vi "Example Three Stage.vi"() -> ()   [LabVIEW 2019]
uses:
  Class/Controller/Controller.lvclass
  <vilib>/Platform/TimedLoop/XDataNode/timing_clust.ctl
  <vilib>/Platform/TimedLoop/XDataNode/nitl_modes.ctl
  <vilib>/Platform/TimedLoop/XDataNode/wakeup.ctl
  <vilib>/platform/TimedLoop/XDataNode/XDataNode.xnode
  <vilib>/Platform/TimedLoop/XDataNode/XDNodeRunTimeDep.lvlib
panel:
  in  "Tab Control 3":enum32{"Motion", "Settings"}(tab)
  in  "Zero Output 3":bool
  in  "Go to Home 3":bool
  in  "Scan Right 3":bool
  in  "Scan Left 3":bool
  in  "Continue 3":bool
  in  "Stop 3":bool
  in  "Make Step Right 3":bool
  in  "Step Size \n[selected units] 3":dbl=1.0 format="%#.2f"
  in  "Make Step Left 3":bool
  in  "Desired Speed \n[1µm/s or 0,01deg /s] 3":dbl=10000.0 format="%#.2f"
  in  "Desired Position \n[selected units] 3":dbl format="%#.2f"
  in  "Find Index 3":bool
  in  "Reset 3":bool
  out "Desired Position\n[selected units] 3":dbl
  out "Encoder position \n[selected units] 3":dbl
  out "Waveform Chart 3":dbl(graph)=-0.078
  out "Status Info 3":T1
  out "StatusBits 3":T2
  in  "Working Units 3":string(combo)="1000000"
  in  "Axis Resolution 3":string(combo)="312,5"
  in  "Axis Letter 3":string="Z"
  in  "Tab Control 2":enum32{"Motion", "Settings"}(tab)
  in  "Zero Output 2":bool
  in  "Go to Home 2":bool
  in  "Scan Right 2":bool
  in  "Scan Left 2":bool
  in  "Continue 2":bool
  in  "Stop 2":bool
  in  "Make Step Right 2":bool
  in  "Step Size \n[selected units] 2":dbl=1.0 format="%#.2f"
  in  "Make Step Left 2":bool
  in  "Desired Speed \n[1µm/s or 0,01deg /s] 2":dbl=10000.0 format="%#.2f"
  in  "Desired Position \n[selected units] 2":dbl format="%#.2f"
  in  "Find Index 2":bool
  in  "Reset 2":bool
  out "Desired Position\n[selected units] 2":dbl
  out "Encoder position \n[selected units] 2":dbl
  out "Waveform Chart 2":dbl(graph)=-0.078
  out "Status Info 2":T1
  out "StatusBits 2":T2
  out "Desired Position\n[selected units]":dbl
  out "Encoder position \n[selected units]":dbl
  in  "Tab Control":enum32{"Motion", "Settings"}(tab)
  in  "Zero Output":bool
  in  "Go to Home":bool
  in  "Scan Right":bool
  in  "Scan Left":bool
  in  "Continue":bool
  in  "Stop":bool
  in  "Make Step Right":bool
  in  "Step Size \n[selected units]":dbl=1.0 format="%#.2f"
  in  "Make Step Left":bool
  in  "Desired Speed \n[1µm/s or 0,01deg /s]":dbl=10000.0 format="%#.2f"
  in  "Desired Position \n[selected units]":dbl format="%#.2f"
  in  "Find Index":bool
  in  "Reset":bool
  out "error out":errorcluster
  in  "Working Units 2":string(combo)="1000000"
  in  "Working Units":string(combo)="1000000"
  out "StatusBits":T2
  out "Status Info":T1
  in  "Axis Resolution 2":string(combo)="312,5"
  in  "Axis Letter 2":string="Y"
  in  "Axis Resolution":string(combo)="312,5"
  in  "Axis Letter":string="X"
  in  "Baudrate":u32=9600
  in  "COM Port":refnum<visa-resource-name>
  in  "Controller.lvclass":refnum<class "Controller.lvclass">
  out "Waveform Chart":dbl(graph)=-0.078
  in  "STOP PROGRAM":bool
  # "Visualization"
  # "Extra information"
  # "READ ME FIRST"
  # "Configuration"
  # "Stage 1"
  # "Driver 1"
  # "Stage 1"
  # "How to run:"
  # "BEFORE RUNNING:"
  # "1, Select COM Port"
  # "2. Select baudrate"
  # "3. For each axis:"
  # "3.1 Specify correct axis name (1 letter)"
  # "3.2 Specify correct resolution"
  # "4. Run VI"
  # "WHEN RUNNING, YOU HAVE TO FIRST PUSH \"FIND INDEX\" FOR EACH STAGE.\nThe stages will start moving and find its position. After that you can control the stages"
  # "Stage 2"
  # "NOTES: Do this only the first time"
  # "1. Replace the settings_default.txt file with\nthe file we provided on a USB stick."
  # "2.    Make sure there are no comments in the\nsettings_default.txt file. ONLY lines like: \"X:DPOS=100\" so NO \"%\" in front or at the end of the line."
  # "Position Information"
  # "Stage 3"
  # "3.  In your settings_default.txt file:\nEvery line that contains SSPD or MSPD: multiply that value with:\n - 1000 for a lineair stage \n - 100 for a rotating stage"
  # "STOP BUTTON"
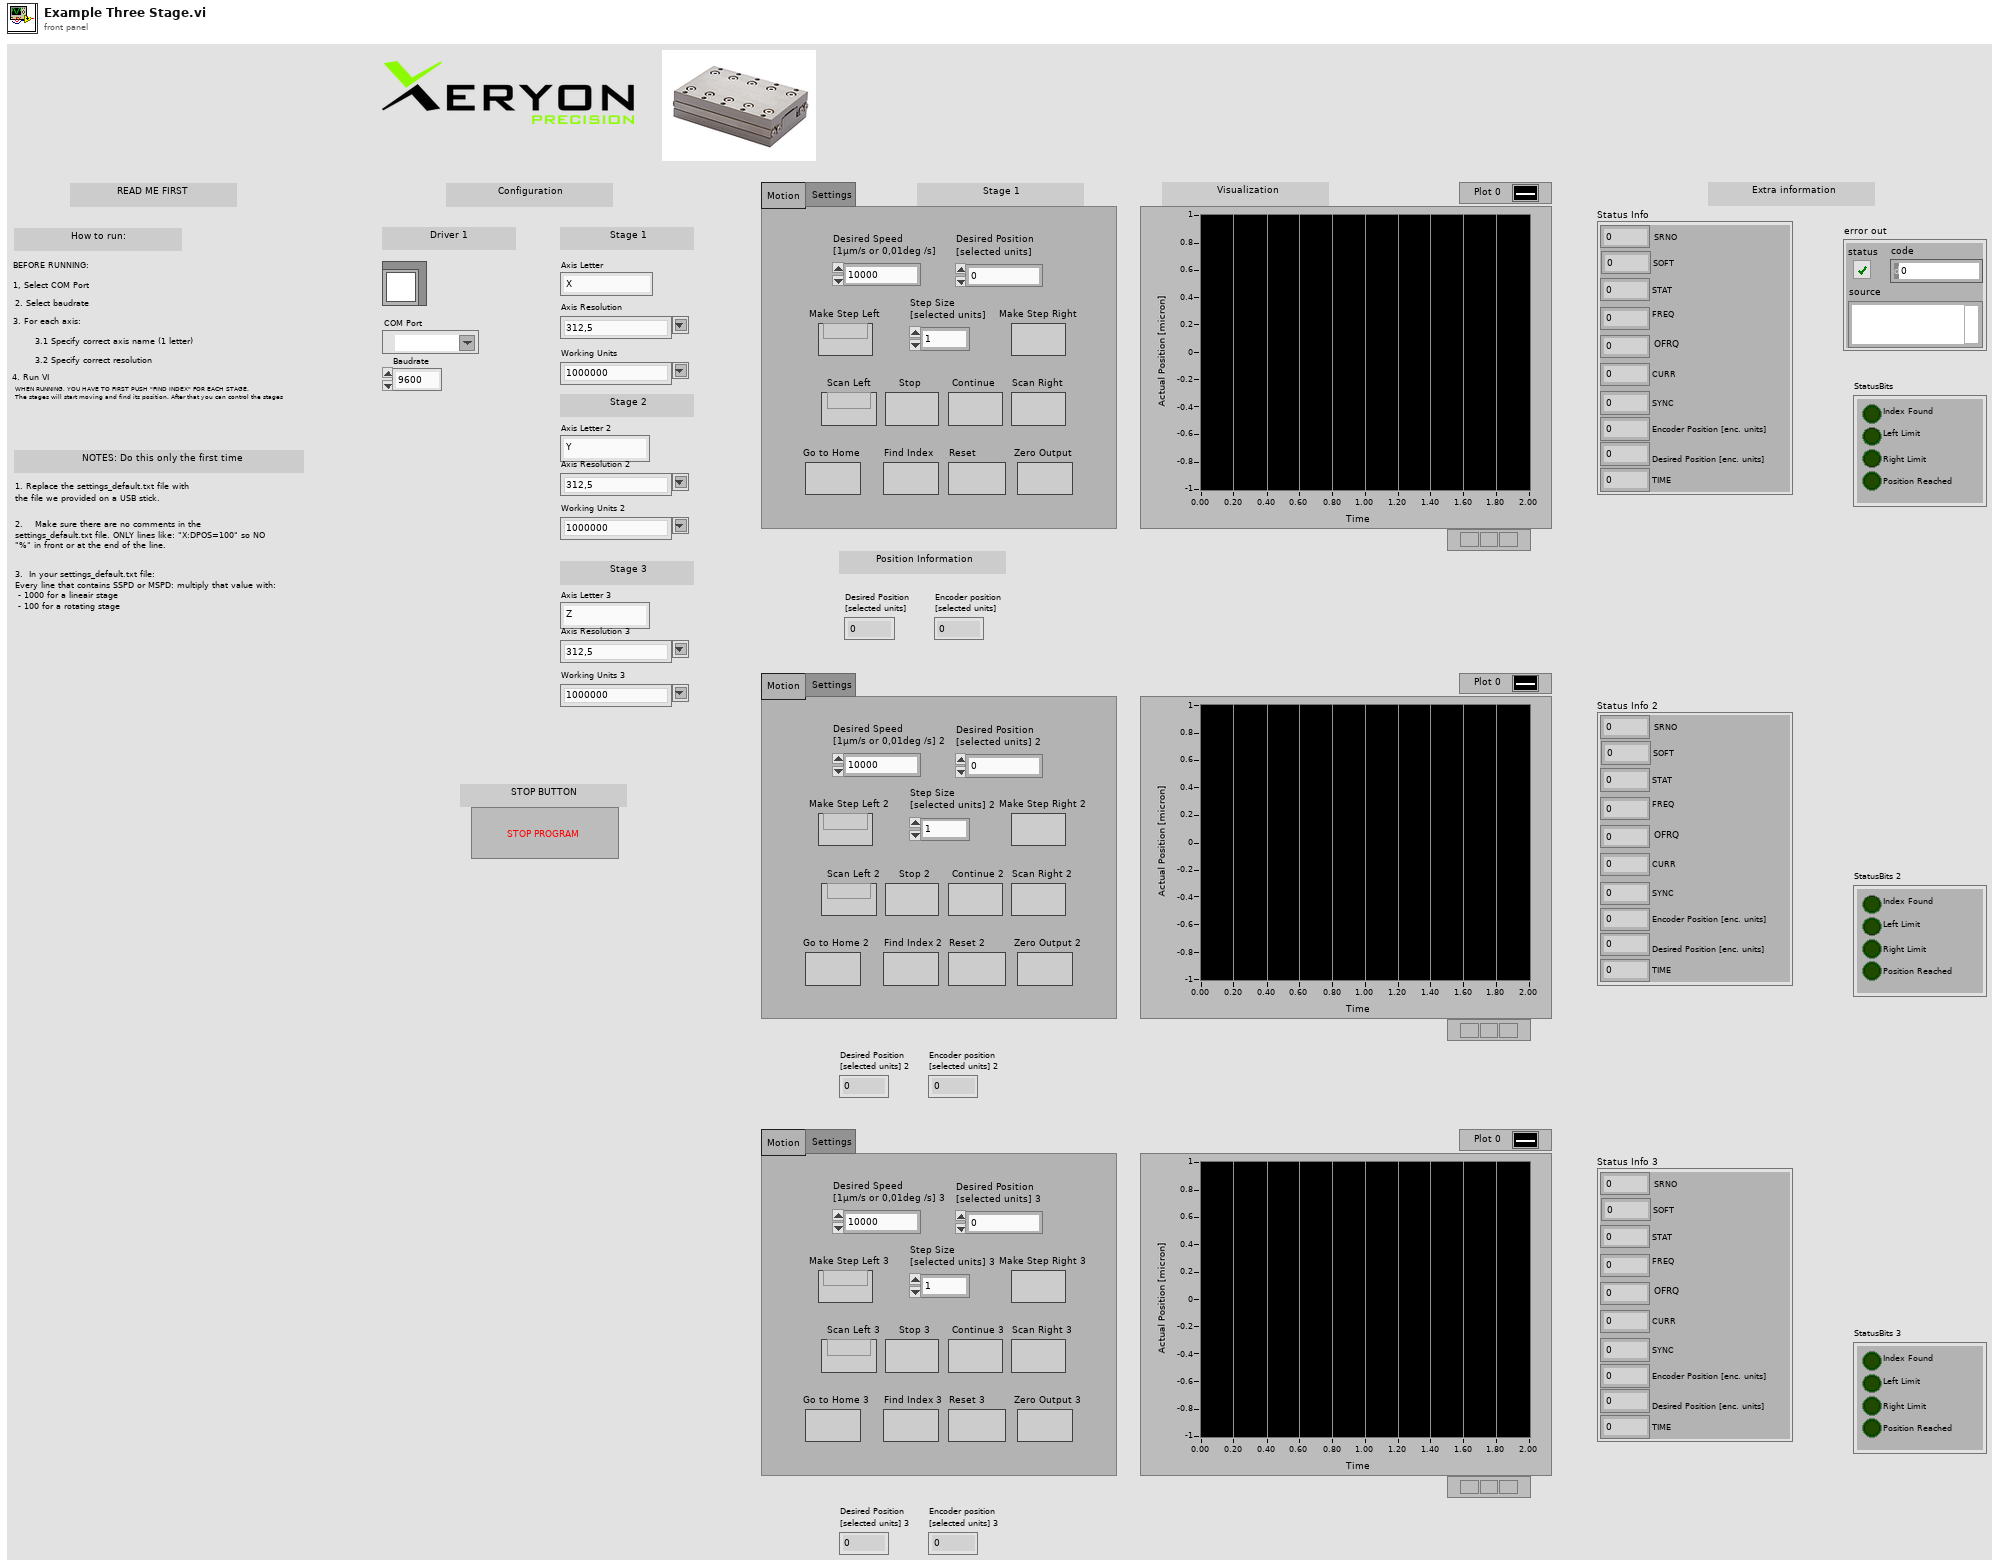
[diagram p1: front panel]
types:
  T1 = cluster{"SRNO":dbl, "SOFT":dbl, "STAT":dbl, "FREQ":dbl, "OFRQ":dbl, "CURR":dbl, "SYNC":dbl, "Encoder Position [enc. units]":dbl, "Desired Position [enc. units]":dbl, "TIME":dbl}
  T2 = cluster{"Index Found":bool, "Left Limit":bool, "Right Limit":bool, "Position Reached":bool}
  T3 = typedef "XDNodeRunTimeDep.lvlib/timing_clust.ctl" = cluster{"Expected End [f-1]":u64, "Actual End [f-1]":u64, "Finished Late? [f-1]":bool, "Expected End [i-1]":u64, "Actual End [i-1]":u64, "Finished Late? [i-1]":bool, "Expected Start [i]":u64, "Actual Start [i]":u64, "Expected Start [f]":u64, "Actual Start [f]":u64, "Source Name":string, "Structure Name":string, "Period":i64, "Deadline":i64, "Offset":i64, "Start":i64, "Priority":i32, "Timeout":i32, "Mode":T4, "Wakeup Reason":T5, "Error":errorcluster, "Source Type":string, "Secondary Source Type":string, "Global End Time":u64, "Global Start Time":u64, "Frame Duration":u64, "Iteration Duration":u64, "Assigned CPU":i32, "I/O Scan Engine Mode":u32}
  T4 = typedef "XDNodeRunTimeDep.lvlib/nitl_modes.ctl" = enum32{"No Change", "Process missed periods, maintain original phase", "Discard missed periods, maintain original phase", "Process missed periods, ignore original phase", "Discard missed periods, ignore original phase"}
  T5 = typedef "XDNodeRunTimeDep.lvlib/wakeup.ctl" = enum32{"Normal", "Aborted", "Asynchronous wakeup", "Timing source error", "Timed loop error", "Timeout"}
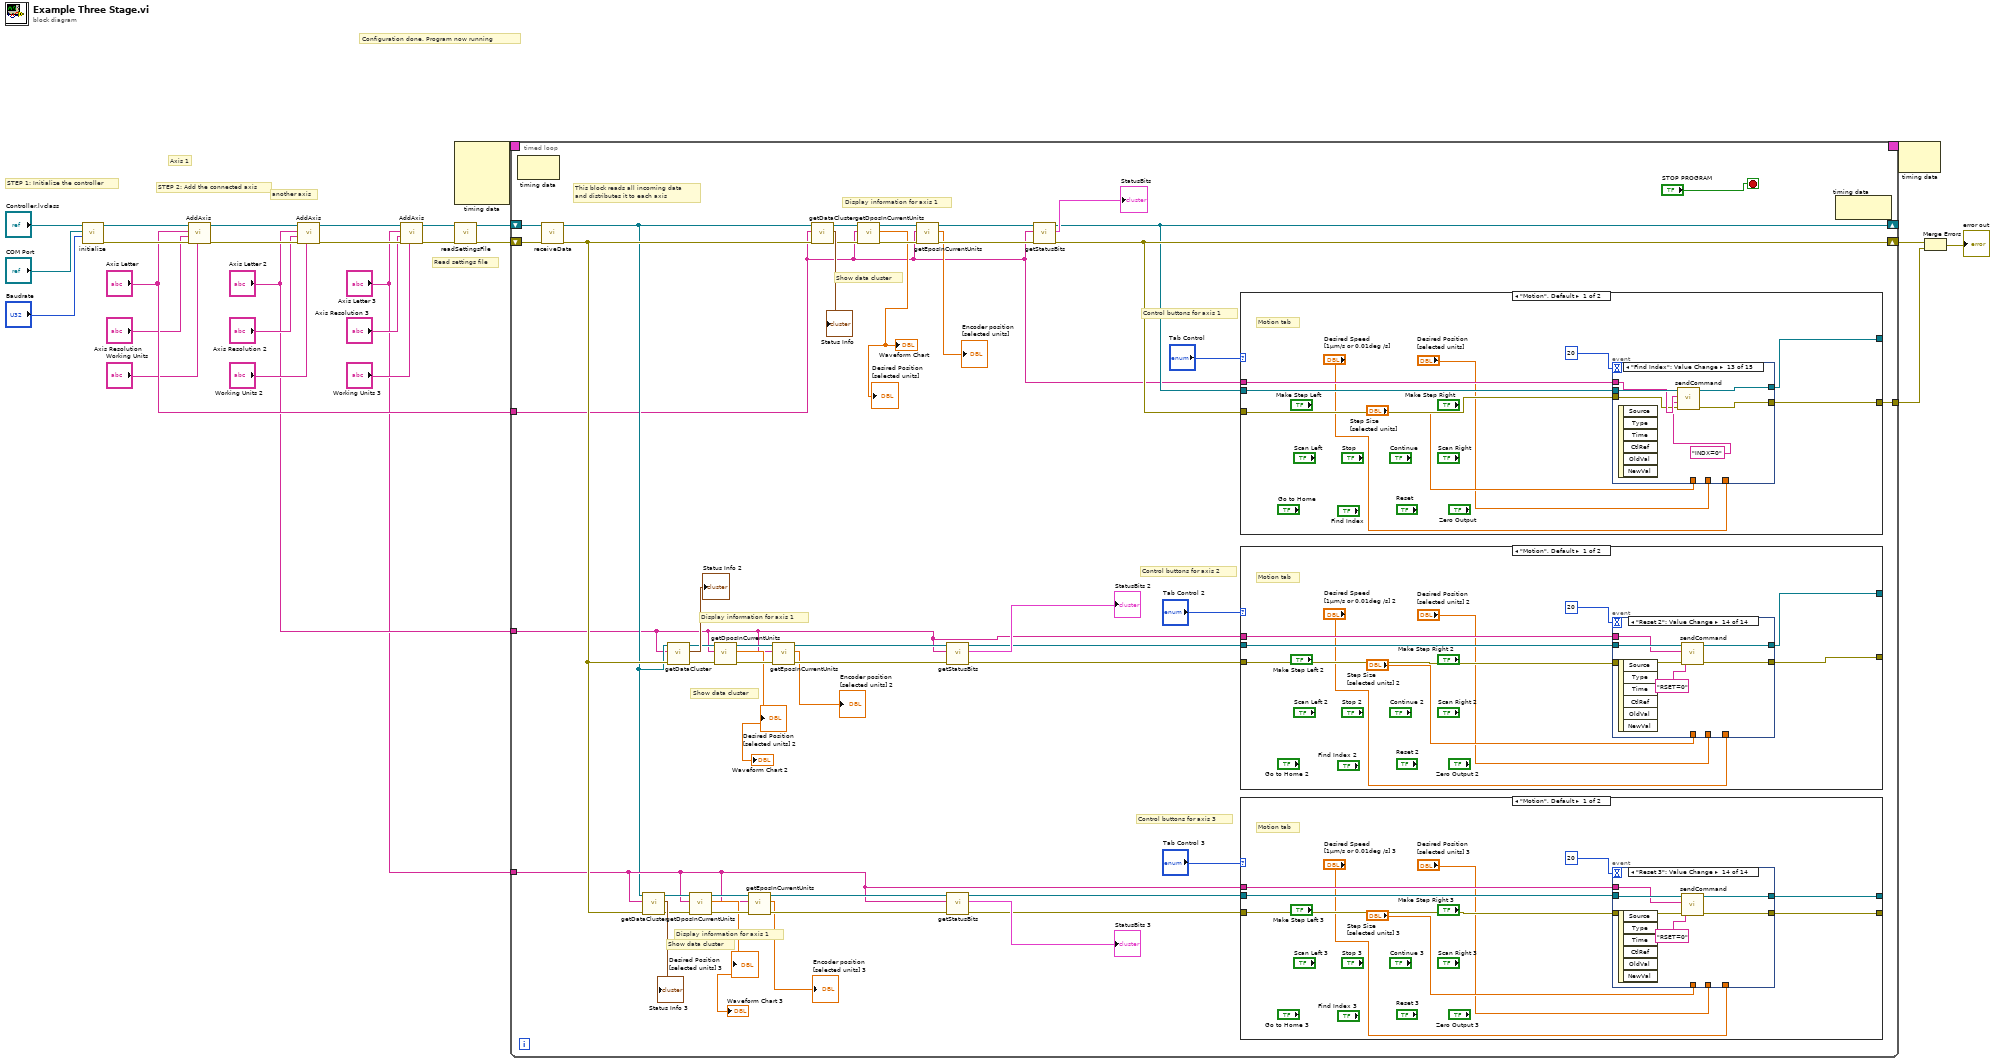
[diagram p0: block diagram]
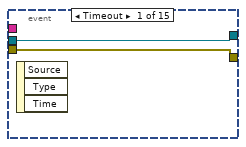
[diagram p2: hidden frame]
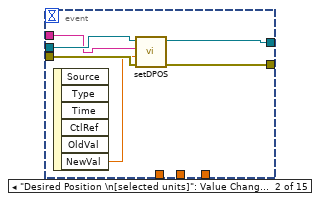
[diagram p3: hidden frame]
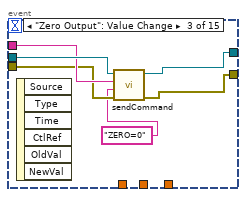
[diagram p4: hidden frame]
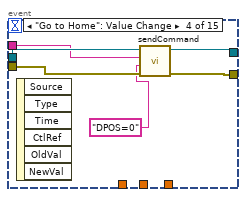
[diagram p5: hidden frame]
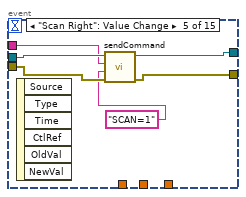
[diagram p6: hidden frame]
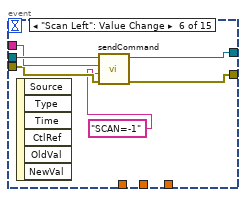
[diagram p7: hidden frame]
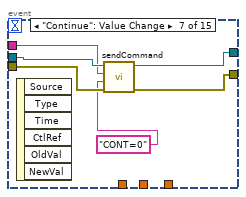
[diagram p8: hidden frame]
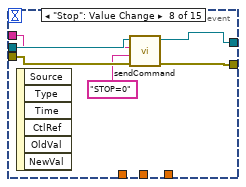
[diagram p9: hidden frame]
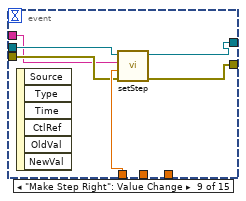
[diagram p10: hidden frame]
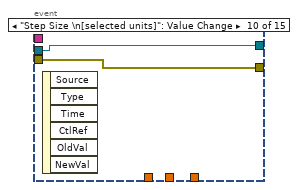
[diagram p11: hidden frame]
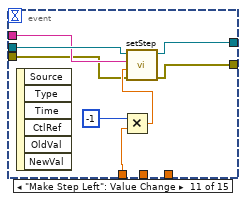
[diagram p12: hidden frame]
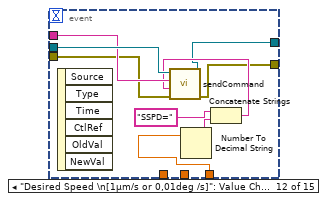
[diagram p13: hidden frame]
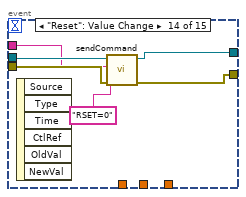
[diagram p14: hidden frame]
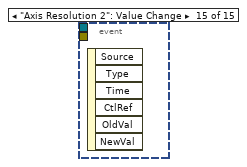
[diagram p15: hidden frame]
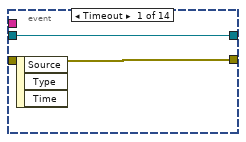
[diagram p17: hidden frame]
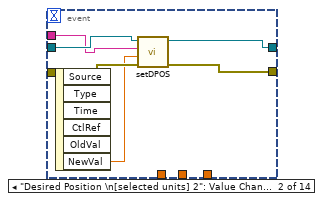
[diagram p18: hidden frame]
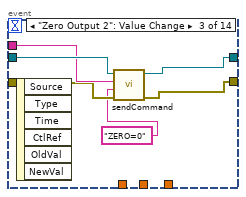
[diagram p19: hidden frame]
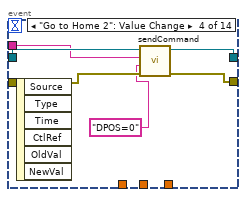
[diagram p20: hidden frame]
diagram:
  # "Axis 1"
  # "Configuration done. Program now running"
  # "Read settings file"
  # "another axis"
  # "STEP 2: Add the connected axis"
  # "STEP 1: Initialize the controller"
  n1 = call-dynamic "initialize.vi"("Baudrate"="Baudrate", "COM Port"="COM Port", "Controller in"="Controller.lvclass") -> ("error out"=w26:errorcluster, "Controller out"=w27:refnum<class "Controller.lvclass">)  [unwired: 7 in]
  n2 = call-dynamic "AddAxis.vi"("Units"="Working Units", "error in (no error)"=w26, "Encoder Resolution"="Axis Resolution", "Axis Letter"="Axis Letter", "Controller in"=w27) -> ("error out"=w24:errorcluster, "Controller out"=w25:refnum<class "Controller.lvclass">)  [unwired: 5 in]
  n3 = call-dynamic "AddAxis.vi"("Units"="Working Units 2", "error in (no error)"=w24, "Encoder Resolution"="Axis Resolution 2", "Axis Letter"="Axis Letter 2", "Controller in"=w25) -> ("error out"=w11:errorcluster, "Controller out"=w12:refnum<class "Controller.lvclass">)  [unwired: 5 in]
  n4 = call-dynamic "AddAxis.vi"("Units"="Working Units 3", "error in (no error)"=w11, "Encoder Resolution"="Axis Resolution 3", "Axis Letter"="Axis Letter 3", "Controller in"=w12) -> ("error out"=w19:errorcluster, "Controller out"=w21:refnum<class "Controller.lvclass">)  [unwired: 5 in]
  n5 = node-c288() -> (w9:T3)  [unwired: 4 in]
  n6 = call-dynamic "readSettingsFile.vi"("error in (no error)"=w19, "Controller in"=w21) -> ("error out"=w18:errorcluster, "Controller out"=w20:refnum<class "Controller.lvclass">)  [unwired: 8 in]
  n7 = timed-loop {
    shift-right: [w29] -> _
    shift-left: w20 -> [w75]
    tunnel: "Axis Letter" -> [w28]
    shift-right: [w61] -> w7
    shift-left: w18 -> [w64]
    timing: w9 -> [_]
    timing-out: [_] -> w8
    tunnel: [w60] -> w6
    tunnel: "Axis Letter 2" -> [w30]
    tunnel: "Axis Letter 3" -> [w32]
    stop <- "STOP PROGRAM" stop-if-true
    # "Control buttons for axis 3"
    # "Display information for axis 1"
    # "Show data cluster"
    # "Control buttons for axis 2"
    # "Display information for axis 1"
    # "Show data cluster"
    # "Control buttons for axis 1"
    # "Display information for axis 1"
    # "Show data cluster"
    # "This block reads all incoming data\nand distributes it to each axis"
    n8 = node-c288() -> ()  [unwired: 1 in, 1 out]
    n9 = call-dynamic "receiveData.vi"("error in (no error)"=w64, "Controller in"=w75) -> ("error out"=w33:errorcluster, "Controller out"=w31:refnum<class "Controller.lvclass">)  [unwired: 7 in, 1 out]
    n10 = call-dynamic "getDataCluster.vi"("error in (no error)"=w33, "Axis Letter"=w32, "Controller in"=w31) -> ("error out"=w41:errorcluster, "Information"=→"Status Info 3":T1, "Controller out"=w44:refnum<class "Controller.lvclass">)  [unwired: 6 in]
    n11 = call-dynamic "getDataCluster.vi"("error in (no error)"=w33, "Axis Letter"=w30, "Controller in"=w31) -> ("error out"=w54:errorcluster, "Information"=→"Status Info 2":T1, "Controller out"=w57:refnum<class "Controller.lvclass">)  [unwired: 6 in]
    n12 = call-dynamic "getDposInCurrentUnits.vi"("error in (no error)"=w41, "Axis Letter"=w32, "Controller in"=w44) -> ("error out"=w40:errorcluster, "DPOS In Current Units"=→"Waveform Chart 3" →"Desired Position\n[selected units] 3":dbl, "Controller out"=w43:refnum<class "Controller.lvclass">)  [unwired: 6 in]
    n13 = call-dynamic "getDposInCurrentUnits.vi"("error in (no error)"=w54, "Axis Letter"=w30, "Controller in"=w57) -> ("error out"=w53:errorcluster, "DPOS In Current Units"=→"Waveform Chart 2" →"Desired Position\n[selected units] 2":dbl, "Controller out"=w56:refnum<class "Controller.lvclass">)  [unwired: 6 in]
    n14 = call-dynamic "getEposInCurrentUnits.vi"("error in (no error)"=w40, "Axis Letter"=w32, "Controller in"=w43) -> ("error out"=w39:errorcluster, "EPOS In Current Units"=→"Encoder position \n[selected units] 3":dbl, "Controller out"=w42:refnum<class "Controller.lvclass">)  [unwired: 6 in]
    n15 = call-dynamic "getEposInCurrentUnits.vi"("error in (no error)"=w53, "Axis Letter"=w30, "Controller in"=w56) -> ("error out"=w52:errorcluster, "EPOS In Current Units"=→"Encoder position \n[selected units] 2":dbl, "Controller out"=w55:refnum<class "Controller.lvclass">)  [unwired: 6 in]
    n16 = call-dynamic "getDataCluster.vi"("error in (no error)"=w33, "Axis Letter"=w28, "Controller in"=w31) -> ("error out"=w69:errorcluster, "Information"=→"Status Info":T1, "Controller out"=w72:refnum<class "Controller.lvclass">)  [unwired: 6 in]
    n17 = call-dynamic "getDposInCurrentUnits.vi"("error in (no error)"=w69, "Axis Letter"=w28, "Controller in"=w72) -> ("error out"=w68:errorcluster, "DPOS In Current Units"=→"Waveform Chart" →"Desired Position\n[selected units]":dbl, "Controller out"=w71:refnum<class "Controller.lvclass">)  [unwired: 6 in]
    n18 = call-dynamic "getEposInCurrentUnits.vi"("error in (no error)"=w68, "Axis Letter"=w28, "Controller in"=w71) -> ("error out"=w67:errorcluster, "EPOS In Current Units"=→"Encoder position \n[selected units]":dbl, "Controller out"=w70:refnum<class "Controller.lvclass">)  [unwired: 6 in]
    n19 = call-dynamic "getStatusBits.vi"("error in (no error)"=w52, "Axis Letter"=w30, "Controller in"=w55) -> ("error out"=w47:errorcluster, "StatusBits"=→"StatusBits 2":T2, "Controller out"=w48:refnum<class "Controller.lvclass">)  [unwired: 6 in]
    n20 = call-dynamic "getStatusBits.vi"("error in (no error)"=w39, "Axis Letter"=w32, "Controller in"=w42) -> ("error out"=w34:errorcluster, "StatusBits"=→"StatusBits 3":T2, "Controller out"=w35:refnum<class "Controller.lvclass">)  [unwired: 6 in]
    n21 = call-dynamic "getStatusBits.vi"("error in (no error)"=w67, "Axis Letter"=w28, "Controller in"=w70) -> ("error out"=w61:errorcluster, "StatusBits"=→"StatusBits":T2, "Controller out"=w29:refnum<class "Controller.lvclass">)  [unwired: 6 in]
    n22 = case shown="\"Motion\", Default" "Tab Control" {
      tunnel: w29 -> [w86 w168]
      tunnel: w61 -> [w85 w169]
      tunnel: [w84 w168] -> _
      tunnel: [w83 w169] -> w60
      tunnel: w28 -> [w81 _]
      frame "Motion", Default {
        # "Motion tab"
        n23 = event shown="[12] \"Find Index\": Value Change" {
          selector: _ -> [_ _ _ _ _ _ _ _ _ _ _ _ _ _ _]
          dyn-events: _ -> [_ _ _ _ _ _ _ _ _ _ _ _ _ _ _]
          timeout: 20 -> [_ _ _ _ _ _ _ _ _ _ _ _ _ _ _]
          tunnel: w86 -> [w88 w94 w100 w106 w112 w118 w124 w130 w134 w138 w144 w155 w161 w167 _]
          tunnel: w85 -> [w87 w93 w98 w104 w110 w116 w122 w128 w135 w137 w141 w153 w159 w166 _]
          tunnel: [w88 w91 w96 w101 w108 w114 w120 w126 w132 w138 w139 w147 w157 w163 _] -> w84
          tunnel: [w87 w92 w97 w103 w109 w115 w121 w127 w131 w137 w140 w148 w158 w162 _] -> w83
          tunnel: w81 -> [_ w89 w99 w105 w111 w117 w123 w129 w133 _ w143 w154 w160 w165 _]
          tunnel: "Step Size \n[selected units]" -> [_ _ _ _ _ _ _ _ w136 _ w145 _ _ _ _]
          tunnel: "Desired Position \n[selected units]" -> [_ _ _ _ _ _ _ _ _ _ _ _ _ _ _]
          tunnel: "Desired Speed \n[1µm/s or 0,01deg /s]" -> [_ _ _ _ _ _ _ _ _ _ _ w152 _ _ _]
          event Timeout {
            n24 = event-data() -> ()  [unwired: 1 in, 3 out]
          }
          event "Desired Position \n[selected units]": Value Change {
            n25 = event-data() -> ("NewVal"=w90:dbl)  [unwired: 1 in, 5 out]
            n26 = call-dynamic "setDPOS.vi"("error in (no error)"=w93, "DPOS In Current Units"=w90, "Axis Letter"=w89, "Controller in"=w94) -> ("error out"=w92:errorcluster, "Controller out"=w91:refnum<class "Controller.lvclass">)  [unwired: 6 in]
          }
          event "Zero Output": Value Change {
            n27 = event-data() -> ()  [unwired: 1 in, 6 out]
            n28 = call-dynamic "sendCommand.vi"("error in (no error)"=w98, "Value"="ZERO=0", "Command"=w99, "Controller in"=w100) -> ("error out"=w97:errorcluster, "Controller out"=w96:refnum<class "Controller.lvclass">)  [unwired: 6 in]
          }
          event "Go to Home": Value Change {
            n29 = event-data() -> ()  [unwired: 1 in, 6 out]
            n30 = call-dynamic "sendCommand.vi"("error in (no error)"=w104, "Value"="DPOS=0", "Command"=w105, "Controller in"=w106) -> ("error out"=w103:errorcluster, "Controller out"=w101:refnum<class "Controller.lvclass">)  [unwired: 6 in]
          }
          event "Scan Right": Value Change {
            n31 = event-data() -> ()  [unwired: 1 in, 6 out]
            n32 = call-dynamic "sendCommand.vi"("error in (no error)"=w110, "Value"="SCAN=1", "Command"=w111, "Controller in"=w112) -> ("error out"=w109:errorcluster, "Controller out"=w108:refnum<class "Controller.lvclass">)  [unwired: 6 in]
          }
          event "Scan Left": Value Change {
            n33 = event-data() -> ()  [unwired: 1 in, 6 out]
            n34 = call-dynamic "sendCommand.vi"("error in (no error)"=w116, "Value"="SCAN=-1", "Command"=w117, "Controller in"=w118) -> ("error out"=w115:errorcluster, "Controller out"=w114:refnum<class "Controller.lvclass">)  [unwired: 6 in]
          }
          event "Continue": Value Change {
            n35 = event-data() -> ()  [unwired: 1 in, 6 out]
            n36 = call-dynamic "sendCommand.vi"("error in (no error)"=w122, "Value"="CONT=0", "Command"=w123, "Controller in"=w124) -> ("error out"=w121:errorcluster, "Controller out"=w120:refnum<class "Controller.lvclass">)  [unwired: 6 in]
          }
          event "Stop": Value Change {
            n37 = event-data() -> ()  [unwired: 1 in, 6 out]
            n38 = call-dynamic "sendCommand.vi"("error in (no error)"=w128, "Value"="STOP=0", "Command"=w129, "Controller in"=w130) -> ("error out"=w127:errorcluster, "Controller out"=w126:refnum<class "Controller.lvclass">)  [unwired: 6 in]
          }
          event "Make Step Right": Value Change {
            n39 = event-data() -> ()  [unwired: 1 in, 6 out]
            n40 = call-dynamic "setStep.vi"("error in (no error)"=w135, "Step Value"=w136, "Axis Letter"=w133, "Controller in"=w134) -> ("error out"=w131:errorcluster, "Controller out"=w132:refnum<class "Controller.lvclass">)  [unwired: 6 in]
          }
          event "Step Size \n[selected units]": Value Change {
            n41 = event-data() -> ()  [unwired: 1 in, 6 out]
          }
          event "Make Step Left": Value Change {
            n42 = event-data() -> ()  [unwired: 1 in, 6 out]
            n43 = Multiply(x=-1, y=w145) -> (x*y=w142:dbl)
            n44 = call-dynamic "setStep.vi"("error in (no error)"=w141, "Step Value"=w142, "Axis Letter"=w143, "Controller in"=w144) -> ("error out"=w140:errorcluster, "Controller out"=w139:refnum<class "Controller.lvclass">)  [unwired: 6 in]
          }
          event "Desired Speed \n[1µm/s or 0,01deg /s]": Value Change {
            n45 = event-data() -> ()  [unwired: 1 in, 6 out]
            n46 = Number To Decimal String(number=w152) -> (decimal integer string=w150:string)  [unwired: 1 in]
            n47 = Concatenate Strings("SSPD=", w150) -> (w149:string)
            n48 = call-dynamic "sendCommand.vi"("error in (no error)"=w153, "Value"=w149, "Command"=w154, "Controller in"=w155) -> ("error out"=w148:errorcluster, "Controller out"=w147:refnum<class "Controller.lvclass">)  [unwired: 6 in]
          }
          event "Find Index": Value Change {
            n49 = event-data() -> ()  [unwired: 1 in, 6 out]
            n50 = call-dynamic "sendCommand.vi"("error in (no error)"=w159, "Value"="INDX=0", "Command"=w160, "Controller in"=w161) -> ("error out"=w158:errorcluster, "Controller out"=w157:refnum<class "Controller.lvclass">)  [unwired: 6 in]
          }
          event "Reset": Value Change {
            n51 = event-data() -> ()  [unwired: 1 in, 6 out]
            n52 = call-dynamic "sendCommand.vi"("error in (no error)"=w166, "Value"="RSET=0", "Command"=w165, "Controller in"=w167) -> ("error out"=w162:errorcluster, "Controller out"=w163:refnum<class "Controller.lvclass">)  [unwired: 6 in]
          }
          event "Axis Resolution 2": Value Change {
            n53 = event-data() -> ()  [unwired: 1 in, 6 out]
          }
        }
      }
      frame "Settings" {
      }
    }
    n54 = case shown="\"Motion\", Default" "Tab Control 2" {
      tunnel: w48 -> [w178 w260]
      tunnel: w47 -> [w177 w261]
      tunnel: [w176 w260] -> _
      tunnel: [w175 w261] -> _
      tunnel: w30 -> [w173 _]
      frame "Motion", Default {
        # "Motion tab"
        n55 = event shown="[13] \"Reset 2\": Value Change" {
          selector: _ -> [_ _ _ _ _ _ _ _ _ _ _ _ _ _]
          dyn-events: _ -> [_ _ _ _ _ _ _ _ _ _ _ _ _ _]
          timeout: 20 -> [_ _ _ _ _ _ _ _ _ _ _ _ _ _]
          tunnel: w178 -> [w180 w186 w192 w198 w204 w210 w216 w222 w226 w230 w236 w247 w253 w259]
          tunnel: w177 -> [w179 w185 w190 w196 w202 w208 w214 w220 w227 w229 w233 w245 w251 w258]
          tunnel: [w180 w183 w188 w193 w200 w206 w212 w218 w224 w230 w231 w239 w249 w255] -> w176
          tunnel: [w179 w184 w189 w195 w201 w207 w213 w219 w223 w229 w232 w240 w250 w254] -> w175
          tunnel: w173 -> [_ w181 w191 w197 w203 w209 w215 w221 w225 _ w235 w246 w252 w257]
          tunnel: "Step Size \n[selected units] 2" -> [_ _ _ _ _ _ _ _ w228 _ w237 _ _ _]
          tunnel: "Desired Position \n[selected units] 2" -> [_ _ _ _ _ _ _ _ _ _ _ _ _ _]
          tunnel: "Desired Speed \n[1µm/s or 0,01deg /s] 2" -> [_ _ _ _ _ _ _ _ _ _ _ w244 _ _]
          event Timeout {
            n56 = event-data() -> ()  [unwired: 1 in, 3 out]
          }
          event "Desired Position \n[selected units] 2": Value Change {
            n57 = event-data() -> ("NewVal"=w182:dbl)  [unwired: 1 in, 5 out]
            n58 = call-dynamic "setDPOS.vi"("error in (no error)"=w185, "DPOS In Current Units"=w182, "Axis Letter"=w181, "Controller in"=w186) -> ("error out"=w184:errorcluster, "Controller out"=w183:refnum<class "Controller.lvclass">)  [unwired: 6 in]
          }
          event "Zero Output 2": Value Change {
            n59 = event-data() -> ()  [unwired: 1 in, 6 out]
            n60 = call-dynamic "sendCommand.vi"("error in (no error)"=w190, "Value"="ZERO=0", "Command"=w191, "Controller in"=w192) -> ("error out"=w189:errorcluster, "Controller out"=w188:refnum<class "Controller.lvclass">)  [unwired: 6 in]
          }
          event "Go to Home 2": Value Change {
            n61 = event-data() -> ()  [unwired: 1 in, 6 out]
            n62 = call-dynamic "sendCommand.vi"("error in (no error)"=w196, "Value"="DPOS=0", "Command"=w197, "Controller in"=w198) -> ("error out"=w195:errorcluster, "Controller out"=w193:refnum<class "Controller.lvclass">)  [unwired: 6 in]
          }
          event "Scan Right 2": Value Change {
            n63 = event-data() -> ()  [unwired: 1 in, 6 out]
            n64 = call-dynamic "sendCommand.vi"("error in (no error)"=w202, "Value"="SCAN=1", "Command"=w203, "Controller in"=w204) -> ("error out"=w201:errorcluster, "Controller out"=w200:refnum<class "Controller.lvclass">)  [unwired: 6 in]
          }
          event "Scan Left 2": Value Change {
            n65 = event-data() -> ()  [unwired: 1 in, 6 out]
            n66 = call-dynamic "sendCommand.vi"("error in (no error)"=w208, "Value"="SCAN=-1", "Command"=w209, "Controller in"=w210) -> ("error out"=w207:errorcluster, "Controller out"=w206:refnum<class "Controller.lvclass">)  [unwired: 6 in]
          }
          event "Continue 2": Value Change {
            n67 = event-data() -> ()  [unwired: 1 in, 6 out]
            n68 = call-dynamic "sendCommand.vi"("error in (no error)"=w214, "Value"="CONT=0", "Command"=w215, "Controller in"=w216) -> ("error out"=w213:errorcluster, "Controller out"=w212:refnum<class "Controller.lvclass">)  [unwired: 6 in]
          }
          event "Stop 2": Value Change {
            n69 = event-data() -> ()  [unwired: 1 in, 6 out]
            n70 = call-dynamic "sendCommand.vi"("error in (no error)"=w220, "Value"="STOP=0", "Command"=w221, "Controller in"=w222) -> ("error out"=w219:errorcluster, "Controller out"=w218:refnum<class "Controller.lvclass">)  [unwired: 6 in]
          }
          event "Make Step Right 2": Value Change {
            n71 = event-data() -> ()  [unwired: 1 in, 6 out]
            n72 = call-dynamic "setStep.vi"("error in (no error)"=w227, "Step Value"=w228, "Axis Letter"=w225, "Controller in"=w226) -> ("error out"=w223:errorcluster, "Controller out"=w224:refnum<class "Controller.lvclass">)  [unwired: 6 in]
          }
          event "Step Size \n[selected units] 2": Value Change {
            n73 = event-data() -> ()  [unwired: 1 in, 6 out]
          }
          event "Make Step Left 2": Value Change {
            n74 = event-data() -> ()  [unwired: 1 in, 6 out]
            n75 = Multiply(x=-1, y=w237) -> (x*y=w234:dbl)
            n76 = call-dynamic "setStep.vi"("error in (no error)"=w233, "Step Value"=w234, "Axis Letter"=w235, "Controller in"=w236) -> ("error out"=w232:errorcluster, "Controller out"=w231:refnum<class "Controller.lvclass">)  [unwired: 6 in]
          }
          event "Desired Speed \n[1µm/s or 0,01deg /s] 2": Value Change {
            n77 = event-data() -> ()  [unwired: 1 in, 6 out]
            n78 = Number To Decimal String(number=w244) -> (decimal integer string=w242:string)  [unwired: 1 in]
            n79 = Concatenate Strings("SSPD=", w242) -> (w241:string)
            n80 = call-dynamic "sendCommand.vi"("error in (no error)"=w245, "Value"=w241, "Command"=w246, "Controller in"=w247) -> ("error out"=w240:errorcluster, "Controller out"=w239:refnum<class "Controller.lvclass">)  [unwired: 6 in]
          }
          event "Find Index 2": Value Change {
            n81 = event-data() -> ()  [unwired: 1 in, 6 out]
            n82 = call-dynamic "sendCommand.vi"("error in (no error)"=w251, "Value"="INDX=0", "Command"=w252, "Controller in"=w253) -> ("error out"=w250:errorcluster, "Controller out"=w249:refnum<class "Controller.lvclass">)  [unwired: 6 in]
          }
          event "Reset 2": Value Change {
            n83 = event-data() -> ()  [unwired: 1 in, 6 out]
            n84 = call-dynamic "sendCommand.vi"("error in (no error)"=w258, "Value"="RSET=0", "Command"=w257, "Controller in"=w259) -> ("error out"=w254:errorcluster, "Controller out"=w255:refnum<class "Controller.lvclass">)  [unwired: 6 in]
          }
        }
      }
      frame "Settings" {
      }
    }
    n85 = case shown="\"Motion\", Default" "Tab Control 3" {
      tunnel: w35 -> [w270 w352]
      tunnel: w34 -> [w269 w353]
      tunnel: [w268 w352] -> _
      tunnel: [w267 w353] -> _
      tunnel: w32 -> [w265 _]
      frame "Motion", Default {
        # "Motion tab"
        n86 = event shown="[13] \"Reset 3\": Value Change" {
          selector: _ -> [_ _ _ _ _ _ _ _ _ _ _ _ _ _]
          dyn-events: _ -> [_ _ _ _ _ _ _ _ _ _ _ _ _ _]
          timeout: 20 -> [_ _ _ _ _ _ _ _ _ _ _ _ _ _]
          tunnel: w270 -> [w272 w278 w284 w290 w296 w302 w308 w314 w318 w322 w328 w339 w345 w351]
          tunnel: w269 -> [w271 w277 w282 w288 w294 w300 w306 w312 w319 w321 w325 w337 w343 w350]
          tunnel: [w272 w275 w280 w285 w292 w298 w304 w310 w316 w322 w323 w331 w341 w347] -> w268
          tunnel: [w271 w276 w281 w287 w293 w299 w305 w311 w315 w321 w324 w332 w342 w346] -> w267
          tunnel: w265 -> [_ w273 w283 w289 w295 w301 w307 w313 w317 _ w327 w338 w344 w349]
          tunnel: "Step Size \n[selected units] 3" -> [_ _ _ _ _ _ _ _ w320 _ w329 _ _ _]
          tunnel: "Desired Position \n[selected units] 3" -> [_ _ _ _ _ _ _ _ _ _ _ _ _ _]
          tunnel: "Desired Speed \n[1µm/s or 0,01deg /s] 3" -> [_ _ _ _ _ _ _ _ _ _ _ w336 _ _]
          event Timeout {
            n87 = event-data() -> ()  [unwired: 1 in, 3 out]
          }
          event "Desired Position \n[selected units] 3": Value Change {
            n88 = event-data() -> ("NewVal"=w274:dbl)  [unwired: 1 in, 5 out]
            n89 = call-dynamic "setDPOS.vi"("error in (no error)"=w277, "DPOS In Current Units"=w274, "Axis Letter"=w273, "Controller in"=w278) -> ("error out"=w276:errorcluster, "Controller out"=w275:refnum<class "Controller.lvclass">)  [unwired: 6 in]
          }
          event "Zero Output 3": Value Change {
            n90 = event-data() -> ()  [unwired: 1 in, 6 out]
            n91 = call-dynamic "sendCommand.vi"("error in (no error)"=w282, "Value"="ZERO=0", "Command"=w283, "Controller in"=w284) -> ("error out"=w281:errorcluster, "Controller out"=w280:refnum<class "Controller.lvclass">)  [unwired: 6 in]
          }
          event "Go to Home 3": Value Change {
            n92 = event-data() -> ()  [unwired: 1 in, 6 out]
            n93 = call-dynamic "sendCommand.vi"("error in (no error)"=w288, "Value"="DPOS=0", "Command"=w289, "Controller in"=w290) -> ("error out"=w287:errorcluster, "Controller out"=w285:refnum<class "Controller.lvclass">)  [unwired: 6 in]
          }
          event "Scan Right 3": Value Change {
            n94 = event-data() -> ()  [unwired: 1 in, 6 out]
            n95 = call-dynamic "sendCommand.vi"("error in (no error)"=w294, "Value"="SCAN=1", "Command"=w295, "Controller in"=w296) -> ("error out"=w293:errorcluster, "Controller out"=w292:refnum<class "Controller.lvclass">)  [unwired: 6 in]
          }
          event "Scan Left 3": Value Change {
            n96 = event-data() -> ()  [unwired: 1 in, 6 out]
            n97 = call-dynamic "sendCommand.vi"("error in (no error)"=w300, "Value"="SCAN=-1", "Command"=w301, "Controller in"=w302) -> ("error out"=w299:errorcluster, "Controller out"=w298:refnum<class "Controller.lvclass">)  [unwired: 6 in]
          }
          event "Continue 3": Value Change {
            n98 = event-data() -> ()  [unwired: 1 in, 6 out]
            n99 = call-dynamic "sendCommand.vi"("error in (no error)"=w306, "Value"="CONT=0", "Command"=w307, "Controller in"=w308) -> ("error out"=w305:errorcluster, "Controller out"=w304:refnum<class "Controller.lvclass">)  [unwired: 6 in]
          }
          event "Stop 3": Value Change {
            n100 = event-data() -> ()  [unwired: 1 in, 6 out]
            n101 = call-dynamic "sendCommand.vi"("error in (no error)"=w312, "Value"="STOP=0", "Command"=w313, "Controller in"=w314) -> ("error out"=w311:errorcluster, "Controller out"=w310:refnum<class "Controller.lvclass">)  [unwired: 6 in]
          }
          event "Make Step Right 3": Value Change {
            n102 = event-data() -> ()  [unwired: 1 in, 6 out]
            n103 = call-dynamic "setStep.vi"("error in (no error)"=w319, "Step Value"=w320, "Axis Letter"=w317, "Controller in"=w318) -> ("error out"=w315:errorcluster, "Controller out"=w316:refnum<class "Controller.lvclass">)  [unwired: 6 in]
          }
          event "Step Size \n[selected units] 3": Value Change {
            n104 = event-data() -> ()  [unwired: 1 in, 6 out]
          }
          event "Make Step Left 3": Value Change {
            n105 = event-data() -> ()  [unwired: 1 in, 6 out]
            n106 = Multiply(x=-1, y=w329) -> (x*y=w326:dbl)
            n107 = call-dynamic "setStep.vi"("error in (no error)"=w325, "Step Value"=w326, "Axis Letter"=w327, "Controller in"=w328) -> ("error out"=w324:errorcluster, "Controller out"=w323:refnum<class "Controller.lvclass">)  [unwired: 6 in]
          }
          event "Desired Speed \n[1µm/s or 0,01deg /s] 3": Value Change {
            n108 = event-data() -> ()  [unwired: 1 in, 6 out]
            n109 = Number To Decimal String(number=w336) -> (decimal integer string=w334:string)  [unwired: 1 in]
            n110 = Concatenate Strings("SSPD=", w334) -> (w333:string)
            n111 = call-dynamic "sendCommand.vi"("error in (no error)"=w337, "Value"=w333, "Command"=w338, "Controller in"=w339) -> ("error out"=w332:errorcluster, "Controller out"=w331:refnum<class "Controller.lvclass">)  [unwired: 6 in]
          }
          event "Find Index 3": Value Change {
            n112 = event-data() -> ()  [unwired: 1 in, 6 out]
            n113 = call-dynamic "sendCommand.vi"("error in (no error)"=w343, "Value"="INDX=0", "Command"=w344, "Controller in"=w345) -> ("error out"=w342:errorcluster, "Controller out"=w341:refnum<class "Controller.lvclass">)  [unwired: 6 in]
          }
          event "Reset 3": Value Change {
            n114 = event-data() -> ()  [unwired: 1 in, 6 out]
            n115 = call-dynamic "sendCommand.vi"("error in (no error)"=w350, "Value"="RSET=0", "Command"=w349, "Controller in"=w351) -> ("error out"=w346:errorcluster, "Controller out"=w347:refnum<class "Controller.lvclass">)  [unwired: 6 in]
          }
        }
      }
      frame "Settings" {
      }
    }
    n116 = node-c288() -> ()  [unwired: 1 in, 1 out]
  }
  n117 = node-c288(w8) -> ()  [unwired: 1 out]
  n118 = Merge Errors(w7, w6) -> (→"error out":errorcluster)
